vi "2 HeadingChooser.vi"() -> (2 "Optimal Heading Out":dbl, 3 "Goodness Functions":T3, 10 "Goodness Weightings":T2={"Target Importance"=0.98, "No Sail Importance"=1.0, "Change Importance"=0.2, "Pure Waypoint \nImportance"=0.0, "Pure Wind \nImportance"=0.0} {"Pure Wind \nImportance" min=0.0 step=0.2; "Pure Waypoint \nImportance" min=0.0 step=0.2; "Change Importance" min=0.0 step=0.2; "No Sail Importance" min=0.0 step=0.2; "Target Importance" min=0.0 step=0.2})   [LabVIEW 2011]
doc: "The Heading Chooser VI is responsible for finding the optimal heading for the boat in order to reach the waypoint. It uses fuzzy-logic inspired goodness function logic to choose a heading. Specifically, the VI takes 3 goodness function curves and makes a weighted combination of them, choosing the heading with the highest total goodness.\n\nThis VI does not contain any code that would limit the component goodness functions to just 3 or to the specific ones of 'target', 'no sail', and 'change'. Only the labels would need changing."
uses:
  2 Typedefs/Goodness Fns Indicator.ctl
  2 Typedefs/Goodness Weightings.ctl
  2 Typedefs/tacking attempt.ctl
  2 Classes/Waypoint/Waypoint.lvclass
  2 Globals/2 TuningConstants.vi
  2 Globals/2 Global.vi
panel:
  out "Tacking Attempt":T1
  out "tack start time":timestamp
  out "start of wire":dbl
  out "end of wire":dbl
  out "Latest Optimal Heading":dbl
  # "huh???\nTODO: talk to NI about this"
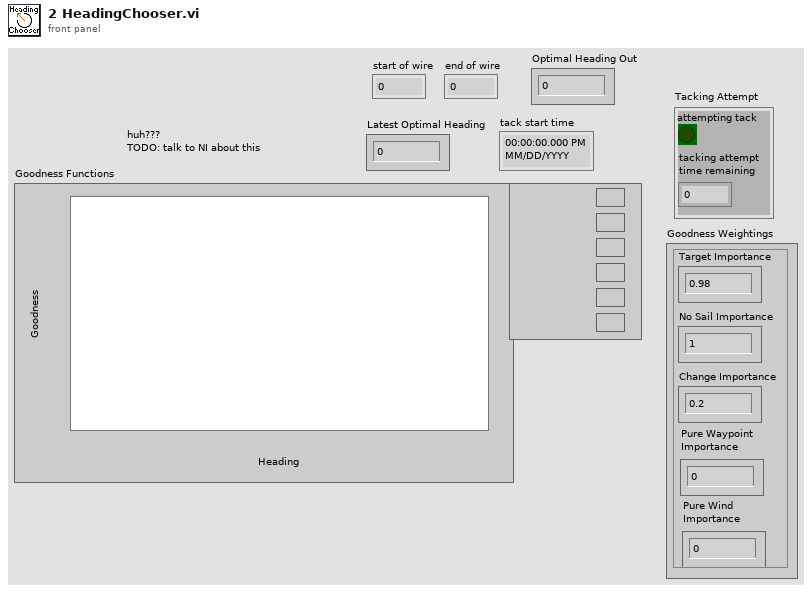
[diagram p1: front panel]
types:
  T1 = typedef "tacking attempt.ctl" = cluster{"attempting tack":bool, "tacking attempt\ntime remaining":dbl}
  T2 = typedef "Goodness Weightings.ctl" = cluster{"Target Importance":dbl, "No Sail Importance":dbl, "Change Importance":dbl, "Pure Waypoint \nImportance":dbl, "Pure Wind \nImportance":dbl}
  T3 = typedef "Goodness Fns Indicator.ctl" = cluster{dbl, dbl, dbl[][]}
  T4 = typedef "UTM Location.ctl" = cluster{"UTM Zone":dbl, "Hemisphere":enum16{"North", "South"}, "East":dbl, "North":dbl}
  T5 = typedef "heading.ctl" = dbl
  T6 = typedef "apparent wind.ctl" = cluster{"Toward Fore":dbl, "Toward Starboard":dbl}
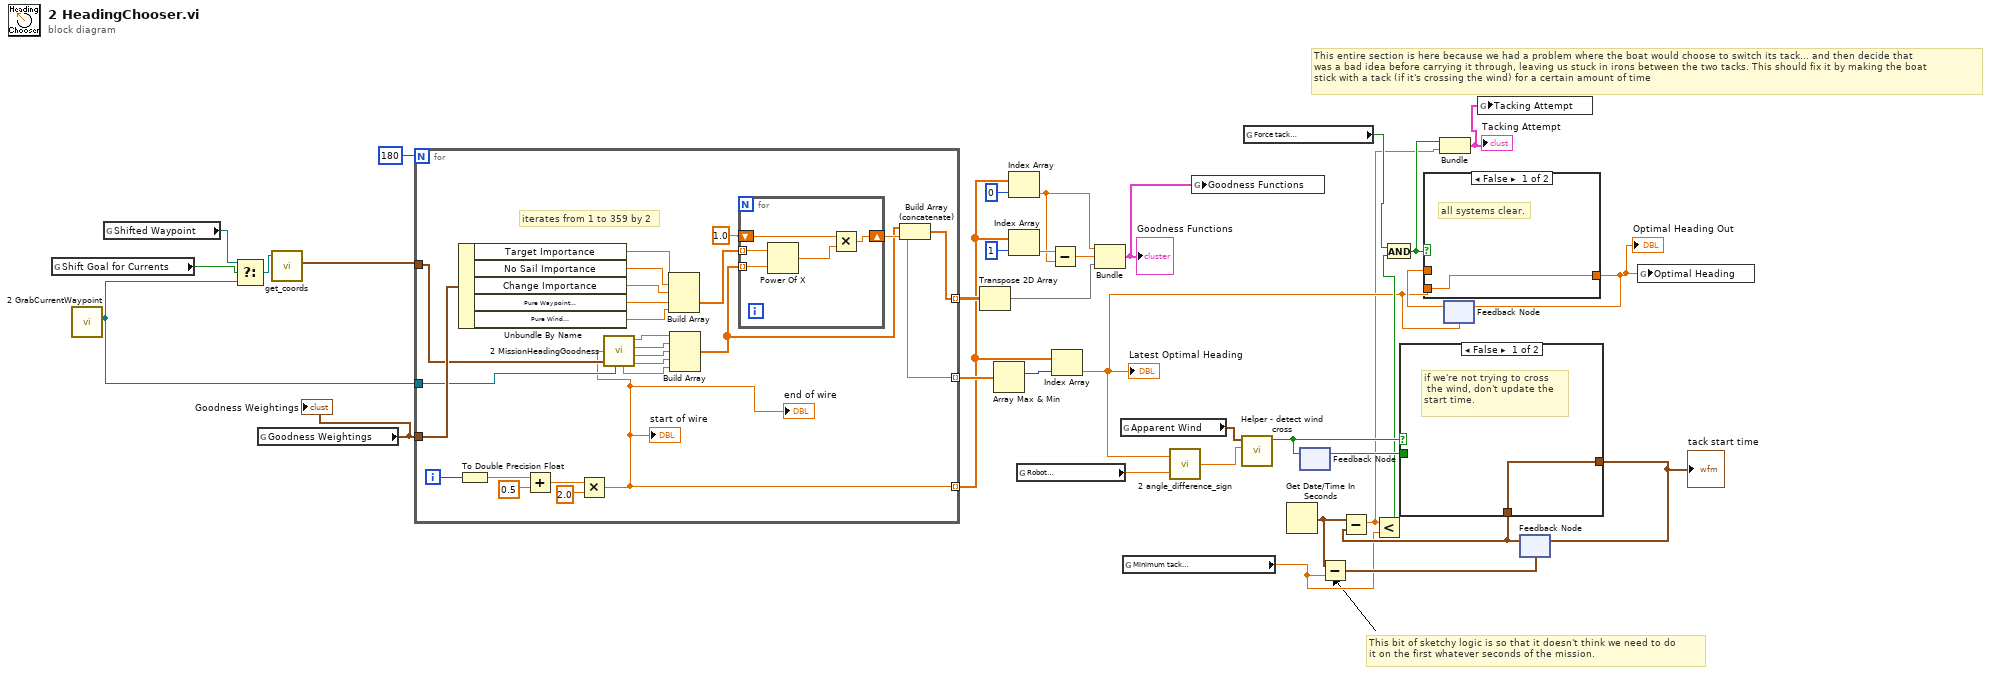
[diagram p0: block diagram]
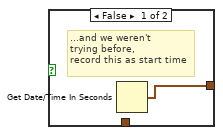
[diagram p4: hidden frame]
diagram:
  # "This entire section is here because we had a problem where the boat would choose to switch its tack... and then decide that\nwas a bad idea before carrying it through, leaving us stuck in irons between the two tacks. This should fix it by making the boat\nstick with a tack (if it's crossing the wind) for a certain amount of time"
  # "This bit of sketchy logic is so that it doesn't think we need to do\nit on the first whatever seconds of the mission."
  n1 = global read "2 Global.vi" "Shift Goal for Currents"() -> (w22:bool)
  n2 = call "2 GrabCurrentWaypoint.vi"() -> ("Current Waypoint"=w21:refnum<class "Waypoint.lvclass">)  [unwired: 11 in]
  n3 = global read "2 Global.vi" "Shifted Waypoint"() -> (w23:refnum<class "Waypoint.lvclass">)
  n4 = Select(t=w23, s=w22, f=w21) -> (s? t:f=w20:refnum<class "Waypoint.lvclass">)
  n5 = global read "2 TuningConstants.vi" "Goodness Weightings"() -> (w30:T2)
  "Goodness Weightings" <- w30
  n6 = call-dynamic "get_coords.vi"("Waypoint in"=w20) -> ("Coords"=w24:T4)  [unwired: 7 in, 3 out]
  n7 = for {
    N: 180 -> [_]
    tunnel: [w55] -> w28 mode=indexing
    tunnel: w30 -> [w59]
    tunnel: w21 -> [w58]
    tunnel: w24 -> [w57]
    tunnel: [w56] -> w29 mode=indexing
    tunnel: [w47] -> w19 mode=indexing
    i -> [w60]
    # "iterates from 1 to 359 by 2"
    n8 = Unbundle By Name(w59) -> ("Target Importance"=w42:dbl, "No Sail Importance"=w43:dbl, "Change Importance"=w44:dbl, "Pure Waypoint \nImportance"=w45:dbl, "Pure Wind \nImportance"=w46:dbl)
    n9 = To Double Precision Float(number=w60) -> (double precision float=w53:dbl)
    n10 = Add(x=w53, y=0.5) -> (x+y=w52:dbl)
    n11 = Multiply(x=w52, y=2.0) -> (x*y=w47:dbl)
    "end of wire" <- w47
    "start of wire" <- w47
    n12 = call "2 MissionHeadingGoodness.vi"("Heading\nto Test"=w47, "Waypoint Location"=w57, "Waypoint in"=w58) -> ("Target Goodness"=w41:dbl, "No-Sail Goodness"=w40:dbl, "Pure Wind Goodness"=w37:dbl, "Direction Change Goodness"=w39:dbl, "Pure Waypoint Goodness"=w38:dbl)  [unwired: 3 in]
    n13 = Build Array(w42, w43, w44, w45, w46) -> (w49:dbl[])
    n14 = Build Array(w41, w40, w39, w38, w37) -> (w48:dbl[])
    n15 = for {
      tunnel: w48 -> [w65] mode=indexing
      tunnel: w49 -> [w64] mode=indexing
      shift-right: [w62] -> w55
      shift-left: 1.0 -> [w61]
      n16 = Power Of X(1:w65, 2:w64) -> (0:w63:dbl)
      n17 = Multiply(x=w61, y=w63) -> (x*y=w62:dbl)
    }
    n18 = Build Array (concatenate)(w48, w55) -> (w56:dbl[])
  }
  n19 = Transpose 2D Array(2D array=w29) -> (transposed array=w25:dbl[][])
  n20 = Array Max & Min(array=w28) -> (max index (indices)=w32:i32)  [unwired: 3 out]
  n21 = Index Array(array=w19, index=0) -> (element=w27:dbl)
  n22 = Index Array(array=w19, index=1) -> (element=w35:dbl)
  n23 = global read "2 Global.vi" "Robot\nHeading"() -> (w17:T5)
  n24 = Subtract(x=w35, y=w27) -> (x-y=w26:dbl)
  n25 = Index Array(array=w19, index=w32) -> (element=w6:dbl)
  "Latest Optimal Heading" <- w6
  n26 = Bundle(w27, w26, w25) -> (w31:cluster{dbl, dbl, dbl[][]})  [unwired: 1 in]
  "Goodness Functions" <- w31
  n27 = global read "2 Global.vi" "Apparent Wind"() -> (w18:T6)
  n28 = global read "2 TuningConstants.vi" "Minimum tack\ntry time?"() -> (w5:dbl)
  n29 = call "2 angle_difference_sign.vi"("Angle 2"=w17, "Angle 1"=w6) -> ("Difference"=w16:dbl)
  n30 = global write "2 Global.vi" "Goodness Functions"(w31) -> ()
  n31 = call "Helper - detect wind cross.vi"("Heading Change"=w16, "Apparent Wind"=w18) -> ("Crossing Wind?"=w15:bool)  [unwired: 9 in]
  n32 = global read "2 TuningConstants.vi" "Force tack\nattempt?"() -> (w4:bool)
  n33 = Get Date/Time In Seconds() -> (seconds since 1Jan1904=w11:timestamp)
  n34 = feedback #1() -> (w14:bool)  [unwired: 1 in]
  n35 = feedback-in #1(w15) -> ()
  n36 = Subtract(x=w11, y=w5) -> (x-y=w10:timestamp)
  n37 = feedback #2(w6) -> (w7:dbl)
  n38 = feedback #3(w10) -> (w12:timestamp)
  n39 = Subtract(x=w11, y=w12) -> (x-y=w2:dbl)
  n40 = Less?(x=w2, y=w5) -> (x < y?=w9:bool)
  n41 = And(x=w4, y=w9) -> (x .and. y?=w3:bool)
  n42 = case shown="False" w15 {
    tunnel: w14 -> [_ w69]
    tunnel: [w66 w68] -> w13
    tunnel: w12 -> [w66 w67]
    frame False {
      # "if we're not trying to cross\n the wind, don't update the\nstart time."
    }
    frame True {
      # "if we're trying to cross the wind..."
      n43 = case shown="True" w69 {
        tunnel: [w70 w71] -> w68
        tunnel: w67 -> [_ w71]
        frame False {
          # "...and we weren't\ntrying before,\nrecord this as start time"
          n44 = Get Date/Time In Seconds() -> (seconds since 1Jan1904=w70:timestamp)
        }
        frame True {
          # "and we were trying to\nbefore, keep counting"
        }
      }
    }
  }
  "tack start time" <- w13
  n45 = case shown="False" w3 {
    tunnel: w6 -> [w72 _]
    tunnel: [w72 w73] -> w8
    tunnel: w7 -> [_ w73]
    frame False {
      # "all systems clear."
    }
    frame True {
      # "if it's been less than 5\nseconds since we started\ntrying to cross the wind,\ndon't let the boat change its\nmind"
    }
  }
  "Optimal Heading Out" <- w8
  n46 = Bundle(w3, w2) -> (w1:cluster{bool, dbl})  [unwired: 1 in]
  "Tacking Attempt" <- w1
  n47 = feedback-in #2(w8) -> ()
  n48 = global write "2 Global.vi" "Tacking Attempt"(w1) -> ()
  n49 = feedback-in #3(w13) -> ()
  n50 = global write "2 Global.vi" "Optimal Heading"(w8) -> ()
